vi "Out of Bounds.vi"(7 "error source vi name":string, 8 "error in (no error)":errorcluster, 9 "length":u64 format="%d bytes", 10 "offset":u64 format="%d bytes", 11 "Pointer in":refnum<class "Pointer.lvclass">) -> (0 "error out":errorcluster, 3 "Pointer out":refnum<class "Pointer.lvclass">)   [LabVIEW 2017, in "Memory Manager.lvlib" / "Pointer.lvclass"]
uses:
  Pointer.lvclass
  Public/Errors.ctl
  Pointer.lvclass/Pointer.ctl
  API/Accessors/Get Size.vi
  Error Building/Get Error Info.vi
  VIs/VIs for Poly/Write U64 into Source.vi
  VIs/Set Error Source.vi
  VIs/Set Error Code.vi
  VIs/Set Error Status.vi
  Constants/Constants.vi
  Constants/Library Name.vi
  VIs/Create Error Cluster.vi
  VIs/VIs for Poly/Create Error Cluster (256B).vi
  Deterministic Error Builder.lvlib
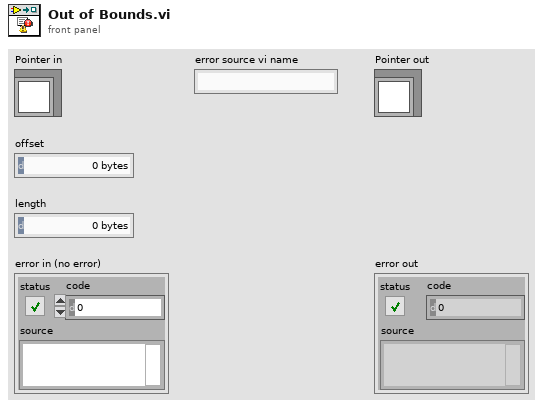
[diagram p1: front panel]
types:
  T1 = typedef "Memory Manager.lvlib/Pointer.lvclass/Errors.ctl" = enum16{"No Error", "Null Pointer", "Out of Bounds", "Buffer Underflow", "Size Mismatch", "Zone"}
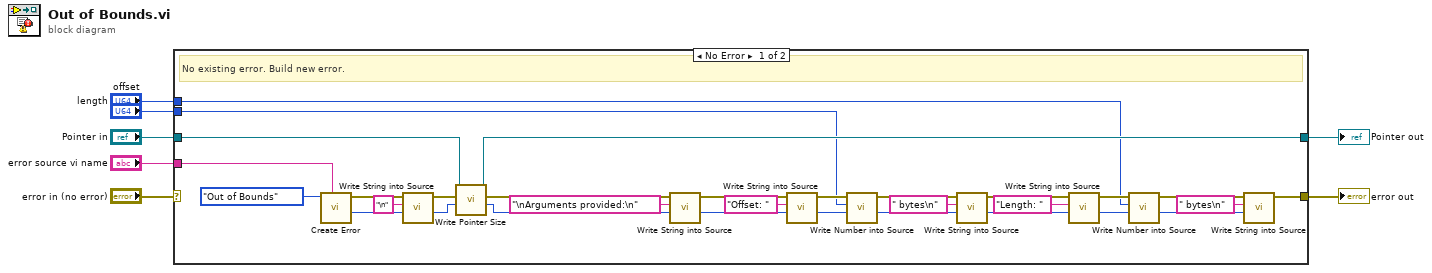
[diagram p0: block diagram]
diagram:
  n1 = case shown="No Error" "error in (no error)" {
    selector: "error in (no error)" -> [_ w40]
    tunnel: [w14 w40] -> w4
    tunnel: "offset" -> [w26 _]
    tunnel: "error source vi name" -> [w30 _]
    tunnel: "Pointer in" -> [w35 w39]
    tunnel: [w34 w39] -> w2
    tunnel: "length" -> [w13 _]
    frame No Error {
      # "No existing error. Build new error."
      n2 = call "Create Error.vi"("source vi name"=w30, "error"=Errors."Out of Bounds") -> ("new offset"=w32:i32, "error out"=w33:errorcluster)  [unwired: 8 in]
      n3 = call "Write String into Source.vi"("offset"=w32, "string"="\n", "error in"=w33) -> ("new offset"=w36:i32, "error out"=w37:errorcluster)  [unwired: 7 in]
      n4 = call "Write Pointer Size.vi"("offset"=w36, "error in"=w37, "Pointer in"=w35) -> ("new offset"=w9:i32, "error out"=w12:errorcluster, "Pointer out"=w34:refnum<class "Pointer.lvclass">)  [unwired: 6 in]
      n5 = call "Write String into Source.vi"("offset"=w9, "string"="\nArguments provided:\n", "error in"=w12) -> ("new offset"=w10:i32, "error out"=w11:errorcluster)  [unwired: 7 in]
      n6 = call "Write String into Source.vi"("offset"=w10, "string"="Offset: ", "error in"=w11) -> ("new offset"=w27:i32, "error out"=w28:errorcluster)  [unwired: 7 in]
      n7 = call-poly "Write Number into Source.vi"("offset"=w27, "value"=w26, "error in"=w28) -> ("new offset"=w23:i32, "error out"=w24:errorcluster)  [unwired: 7 in]
      n8 = call "Write String into Source.vi"("offset"=w23, "string"=" bytes\n", "error in"=w24) -> ("new offset"=w15:i32, "error out"=w16:errorcluster)  [unwired: 7 in]
      n9 = call "Write String into Source.vi"("offset"=w15, "string"="Length: ", "error in"=w16) -> ("new offset"=w20:i32, "error out"=w21:errorcluster)  [unwired: 7 in]
      n10 = call-poly "Write Number into Source.vi"("offset"=w20, "value"=w13, "error in"=w21) -> ("new offset"=w17:i32, "error out"=w18:errorcluster)  [unwired: 7 in]
      n11 = call "Write String into Source.vi"("offset"=w17, "string"=" bytes\n", "error in"=w18) -> ("error out"=w14:errorcluster)  [unwired: 7 in, 1 out]
    }
    frame Error {
      # "Incoming error. Pass through."
    }
  }
  "error out" <- w4
  "Pointer out" <- w2
